vi "AlliGator Special Controls Update.vi"(8 "error in (no error)":errorcluster, 9 "AlliGator Settings List Element":T1, 11 "VI Refnum":refnum<vi>) -> (0 "Error Out":errorcluster, 1 "Message":string, 2 "VI Name":string, 3 "VI Refnum (dup)":refnum<vi>)   [LabVIEW 2021, in "AlliGator Settings.lvlib"]
doc: "Handles update of some Settings controls & indicators as a result of settings changes."
uses:
  AlliGator Settings.lvlib
  AlliGator Settings List.ctl
  Variant/Variant to Data/Variant to Boolean.vi
  Variant/Variant to Data/Variant to DBL.vi
  Variant/Variant to Data/Variant to [String].vi
  Variant/Variant to Data/Variant to I32.vi
  Variant/Variant to Data/Variant to Data.lvlib
  Utilities/Utilities.lvlib
panel:
  in  "Operations Order":u16(ring) caption="Order" items=["Revert", "Smoothen", "Straighten", "Extrapolate", "Normalize", "Background subtraction", "Shift"]
  # "see the AlliGator License on the block diagram (Ctrl+E or Window:Show Block Diagram)"
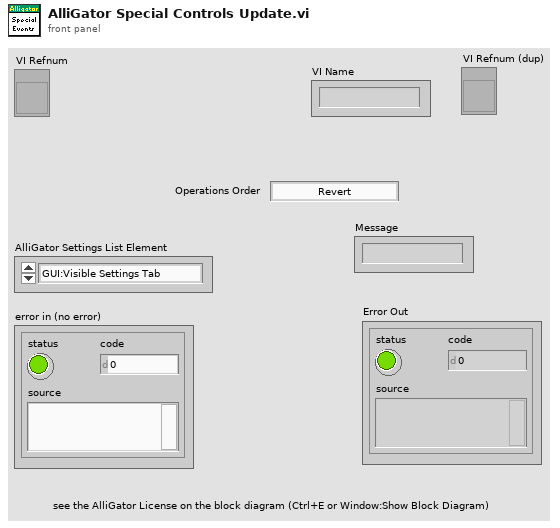
[diagram p1: front panel]
types:
  T1 = typedef "AlliGator Settings.lvlib/AlliGator Settings List.ctl" = enum16{"GUI:Visible Settings Tab", "GUI:Last Run Version", "Source Image:Use Image Histogram for Contrast", "Source Image:Low Count Pixels Rejection Options", "Source Image:High Count Pixels Rejection Options", "Source Image:Use Image Brightness", "Source Image:Blend Overlay with Image Background", "Source Image:Use Fixed ROI Diameter", "Source Image:ROI Diameter", "Source Image:ROI Center Color", "Source Image:Peak Threshold", "Source Image:Intensity Threshold", "Source Image:Image Binning Options", "Source Image:Image Smoothing Options", "Source Image:Image Histogram Active", "Source Image:Invert Binary Mask", "Source Image:Hot Pixel Removal", "Source Image:Overlay Analyzed ROI Center", "Source Image:Auto-Adjust Contrast", "Source Image:Histogram Lower Percentile", "Source Image:Histogram Upper Percentile", "Source Image:Save Source Image", "Source Image:Scale Bar Options", "Source Image:Image Resolution (Pixel Size)", "Source Image:Flatfield Correction", "Source Image:Show Dead Left Columns Correction", "Source Image:Dead Left Columns Correction", "Source Image:Image Pre-Processing Operations Order", "Source Image:Overlay ROI Median", "Source Image:Median Overlay Color", "Data Information:Gate Width", "Data Information:Nanotime Gate Separation", "Data Information:Macrotime Gate Separation", "Data Information:Gate Step", "Data Information:# Gates", "Data Information:Gate Image Exposure", "Data Information:Gate Image Integration", "Data Information:Gates to Skip", "Data Information:Gates to Keep", "Data Information:Define Gates to", "Data Information:Channel Name", "Data Information:Available Channel Names", "Data Information:Channel Arithmetic", "Data Information:Background File Subtraction", "Data Information:Background File", "Data Information:Background Scaling Factor", "Data Information:Background Pile-up Correction", "Data Information:Background Pixel Well Capacity", "Data Information:Laser Period", "Data Information:SYNC Period", "Data Information:Pile-up Correction", "Data Information:Pixel Well Capacity", "Data Information:Dataset Scaling Factor", "Fluorescence Decay_Decay Pre-Processing:Reverse Gates", "Fluorescence Decay_Decay Pre-Processing:Verbose Decay Pre-Processing", "Fluorescence Decay_Decay Pre-Processing:Use Decay Pre-Processing", "Fluorescence Decay_Decay Pre-Processing:Background Subtraction", "Fluorescence Decay_Decay Pre-Processing:Background Definition Range", "Fluorescence Decay_Decay Pre-Processing:Baseline Subtraction Method", "Fluorescence Decay_Decay Pre-Processing:Decay Pre-Processing Operations Order", "Fluorescence Decay_Decay Pre-Processing:Smoothing Parameter", "Fluorescence Decay_Decay Pre-Processing:Shift Decay", "Fluorescence Decay_Decay Pre-Processing:Decay Shift Parameters", "Fluorescence Decay_Decay Pre-Processing:Fold Decay", "Fluorescence Decay_Decay Pre-Processing:# Folds", "Fluorescence Decay_Decay Pre-Processing:1-Normalize Decay", "Fluorescence Decay_Decay Pre-Processing:[0-1]-Normalize Decay", "Fluorescence Decay_Decay Pre-Processing:Smoothen Decay", "Fluorescence Decay_Decay Pre-Processing:Extrapolate Decay", "Fluorescence Decay_Decay Pre-Processing:Use Periodicity", "Fluorescence Decay_Decay Pre-Processing:Use Cursors", "Fluorescence Decay_Decay Pre-Processing:Tail Fraction", "Fluorescence Decay_Decay Pre-Processing:Head Fraction", "Fluorescence Decay_Decay Pre-Processing:Additional Points", "Fluorescence Decay_Decay Pre-Processing:Straighten Decay", "Fluorescence Decay_Decay Pre-Processing:Constant Background", "Fluorescence Decay_Decay Pre-Processing:Pixel-Normalize Decay", "Fluorescence Decay_Advanced Analysis:Extract IRF instead of Decay", "Fluorescence Decay_Advanced Analysis:IRF Extraction Options", "Fluorescence Decay_Advanced Analysis:IRF Optimization Options", "Fluorescence Decay_Advanced Analysis:Square Pulse Options", "Fluorescence Decay_Advanced Analysis:IRF Order", "Fluorescence Decay_Advanced Analysis:IRF Time Constants", "Fluorescence Decay_Advanced Analysis:Wavelet Analysis Options", "Fluorescence Decay_Advanced Analysis:Average Lifetime Options", "Fluorescence Decay_Fit Options:Fit Options", "Fluorescence Decay_Fit Options:Use Legacy Fitting Approach", "Fluorescence Decay_Fit Options:Use Data Information Laser Period", "Fluorescence Decay_Fit Parameters:Displayed Fit Parameters", "Fluorescence Decay_Fit Parameters:Fit Parameter Constraints", "Fluorescence Decay_Fit Parameters:Export Tabulated Results", "Fluorescence Decay_Fit Parameters:MLE Baseline Offset Type", "Fluorescence Decay_Fit Parameters:MLE Baseline Offset", "Fluorescence Decay_Fit Parameters:Guess Parameter Names", "Fluorescence Decay_Fit Parameters:Guess Parameter Values", "Fluorescence Decay_Fit Parameters:Guess Parameters Options", "Fluorescence Decay_Styles:Show Last Decay Only", "Fluorescence Decay_Styles:Decay Graph Color Array", "Fluorescence Decay:Decay Graph Active", "Fluorescence Decay Statistics:Min Peak Value", "Fluorescence Decay Statistics:Reject Low Decay Peak Pixels", "Fluorescence Decay Statistics:Reject High Decay Peak Pixels", "Fluorescence Decay Statistics:Max Peak Value", "Time Traces:Use File Timestamp", "Time Traces:Time Step", "Time Traces:Use Intensity Correction File", "Time Traces:Intensity Correction File", "Phasor Plot:Phasor Plot Smoothing Options", "Phasor Plot:Phasor Plot Size", "Phasor Plot:Phasor Plot Graphics Options", "Phasor Plot:Cumulative Phasor Plot", "Phasor Plot:Use Phasor Brightness", "Phasor Plot:Blend Overlay with Phasor Background", "Phasor Plot:Save Phasor Plot", "Phasor Plot:Show References", "Phasor Plot:Phasor Ratio Decay Range", "Phasor Plot:Exponential Fading", "Phasor Plot:Phasor Ratio Reference Colors", "Phasor Plot:Reference Radius", "Phasor Plot:Show Color Map Vertices", "Phasor Plot:Phasor Plot Active", "Phasor Plot:Phasor Ratio Color Map Type", "Phasor Plot:Phasor Ratio Color Map", "Phasor Plot:Phasor Ratio Display Range", "Phasor Plot:Selected Image ROI(s)", "Phasor Plot:All Image ROIs", "Phasor Plot:Selected Phasor Plot ROI(s)", "Phasor Plot:All Phasor Plot ROIs", "Phasor Plot:Phasor Ratio Color-Coded Quantity", "Phasor Plot:Store Phasor Harmonics", "Phasor Plot:Draw Reference Segment", "Phasor Plot:User-Defined Quantity", "Phasor Graph:Phasor Frequency", "Phasor Graph:Phasor Ratio Type", "Phasor Graph:Pixel-level Phasor Computation", "Phasor Graph:Save Phasor Graph", "Phasor Graph:Phasor Graph Active", "Phasor Graph:Phasor SDV Options", "Phasor Calibration:Use Backup Calibration if needed", "Phasor Graph:Define Shortest Lifetime as", "Phasor Calibration:Backup Calibration Type", "Phasor Calibration:Calibration Type", "Phasor Calibration:Calibration Lifetime", "Phasor Calibration:Calibration Map Algorithm", "Single-Exponential Phasor Locus (SEPL):Gate Parameters", "Single-Exponential Phasor Locus (SEPL):User-defined Gate", "Single-Exponential Phasor Locus (SEPL):User-defined IRF", "Single-Exponential Phasor Locus (SEPL):Phasor Parameters", "Single-Exponential Phasor Locus (SEPL):Decay & IRF Parameters", "Single-Exponential Phasor Locus (SEPL):Display Parameters", "Lifetime Analysis:Decay Analysis Parameters", "Lifetime Analysis:Lifetime Map Active", "Plugins:Python Settings", "Miscellaneous:Verbose Mode", "Miscellaneous:Beep after Script", "Miscellaneous:Saved Image File Format", "Miscellaneous:Exported Gate Image Settings", "Miscellaneous:Include Loading in Timing", "Miscellaneous:Verbose Settings Mode", "Miscellaneous:Histogram Options", "Miscellaneous:Beep on Error", "Miscellaneous:# Logical Processors Used", "Miscellaneous:ROI Description Max Characters", "Miscellaneous:Verbose Error Mode", "Miscellaneous:Transparent Mask Color"}
  T2 = enum16{"Controls & Indicators", "Controls", "Indicators"}
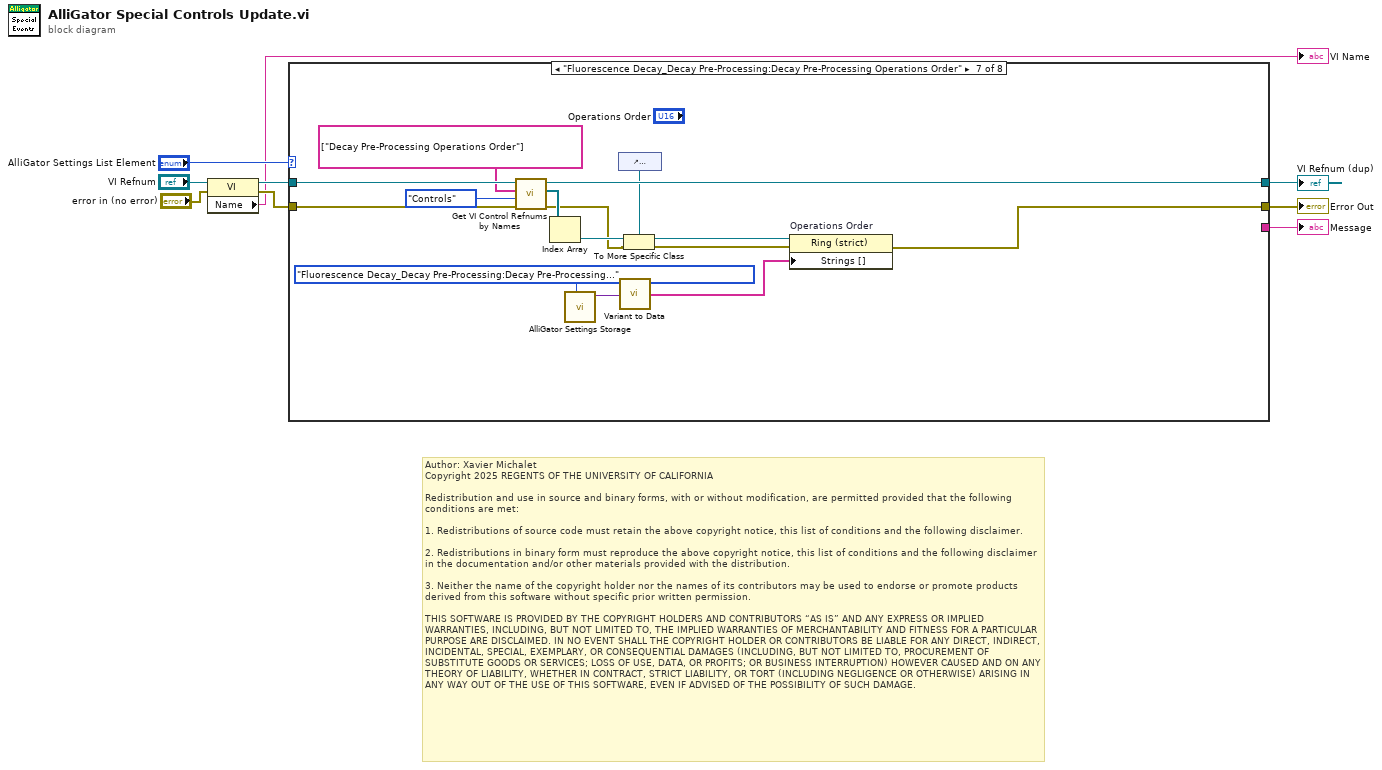
[diagram p0: block diagram]
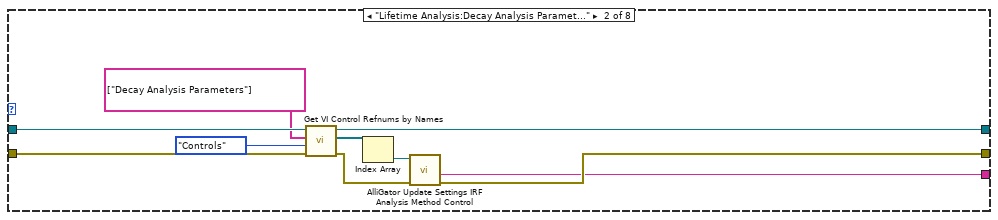
[diagram p3: hidden frame]
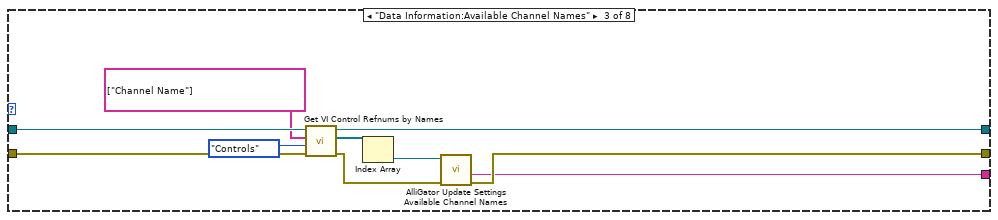
[diagram p4: hidden frame]
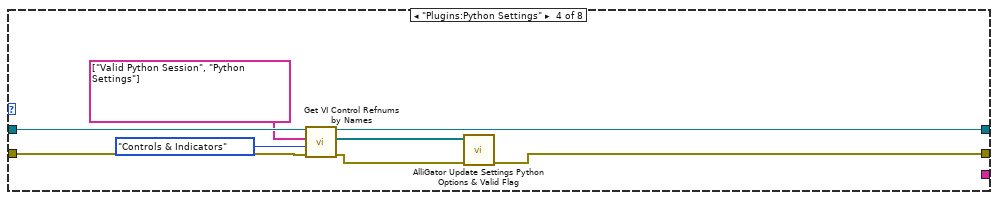
[diagram p5: hidden frame]
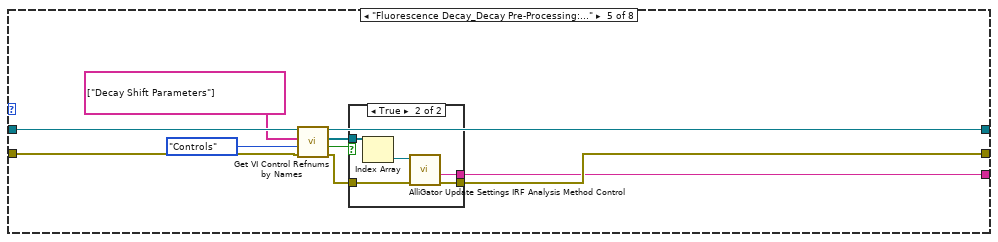
[diagram p6: hidden frame]
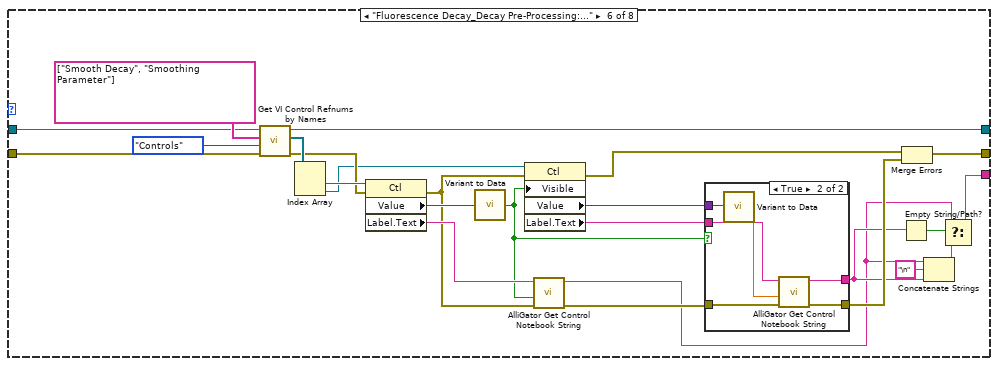
[diagram p8: hidden frame]
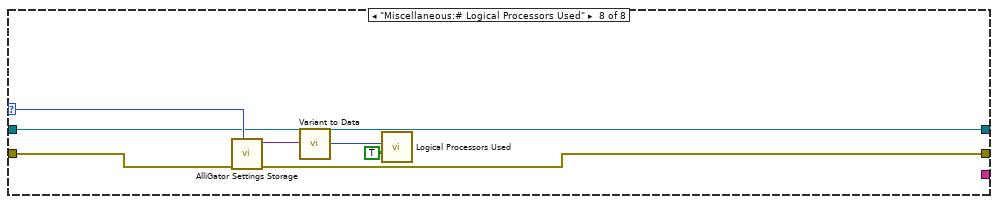
[diagram p10: hidden frame]
diagram:
  # "Author: Xavier Michalet\nCopyright 2025 REGENTS OF THE UNIVERSITY OF CALIFORNIA\n\nRedistribution and use in source and binary forms, with or without modification, are permitted provided that the following conditions are met:\n\n1. Redistributions of source code must retain the above copyright notice, this list of conditions and the following disclaimer.\n\n2. Redistributions in binary form must reproduce the above copyright notice, this list of conditions and the following disclaimer in the documentation and/or other materials provided with the distribution.\n\n3. Neither the name of the copyright holder nor the names of its contributors may be used to endorse or promote products derived from this software without specific prior written permission.\n\nTHIS SOFTWARE IS PROVIDED BY THE COPYRIGHT HOLDERS AND CONTRIBUTORS “AS IS” AND ANY EXPRESS OR IMPLIED WARRANTIES, INCLUDING, BUT NOT LIMITED TO, THE IMPLIED WARRANTIES OF MERCHANTABILITY AND FITNESS FOR A PARTICULAR PURPOSE ARE DISCLAIMED. IN NO EVENT SHALL THE COPYRIGHT HOLDER OR CONTRIBUTORS BE LIABLE FOR ANY DIRECT, INDIRECT, INCIDENTAL, SPECIAL, EXEMPLARY, OR CONSEQUENTIAL DAMAGES (INCLUDING, BUT NOT LIMITED TO, PROCUREMENT OF SUBSTITUTE GOODS OR SERVICES; LOSS OF USE, DATA, OR PROFITS; OR BUSINESS INTERRUPTION) HOWEVER CAUSED AND ON ANY THEORY OF LIABILITY, WHETHER IN CONTRACT, STRICT LIABILITY, OR TORT (INCLUDING NEGLIGENCE OR OTHERWISE) ARISING IN ANY WAY OUT OF THE USE OF THIS SOFTWARE, EVEN IF ADVISED OF THE POSSIBILITY OF SUCH DAMAGE."
  n1 = property class="VI"(reference="VI Refnum", error in="error in (no error)") -> (reference out=w6:refnum<vi>, error out=w4:errorcluster, "Name"=→"VI Name":string)
  n2 = case shown="\"Fluorescence Decay_Decay Pre-Processing:Decay Pre-Processing Operations Order\"" "AlliGator Settings List Element" {
    selector: "AlliGator Settings List Element" -> [_ _ _ _ _ _ _ w109]
    tunnel: w6 -> [w11 w21 w31 w39 w49 w77 w102 w103]
    tunnel: w4 -> [w10 w20 w30 w38 w48 w76 w101 w106]
    tunnel: [w11 w19 w29 w37 w47 w75 w100 w103] -> w2
    tunnel: [w10 w18 w28 w36 w46 w63 w88 w107] -> w8
    tunnel: [_ w17 w27 _ w45 w58 _ _] -> w1
    frame "GUI:Visible Settings Tab", Default {
    }
    frame "Lifetime Analysis:Decay Analysis Parameters" {
      n3 = call "Get VI Control Refnums by Names.vi"("error in"=w20, "Selection"=T2."Controls", "Control Labels"=string[] ["Decay Analysis Parameters"], "VI  Ref"=w21) -> ("error out"=w13:errorcluster, "Ctl Refnums"=w14:refnum<vi>[], "VI  Ref (out)"=w19:refnum<vi>)  [unwired: 4 in, 1 out]
      n4 = Index Array(array=w14) -> (element=w12:refnum<vi>)  [unwired: 1 in]
      n5 = call "AlliGator Update Settings IRF Analysis Method Control.vi"("error in (no error)"=w13, "IRF Analysis Method Refnum"=w12) -> ("error out"=w18:errorcluster, "Message"=w17:string)  [unwired: 8 in]
    }
    frame "Data Information:Available Channel Names" {
      n6 = call "Get VI Control Refnums by Names.vi"("error in"=w30, "Selection"=T2."Controls", "Control Labels"=string[] ["Channel Name"], "VI  Ref"=w31) -> ("error out"=w22:errorcluster, "Ctl Refnums"=w24:refnum<vi>[], "VI  Ref (out)"=w29:refnum<vi>)  [unwired: 4 in, 1 out]
      n7 = Index Array(array=w24) -> (element=w23:refnum<vi>)  [unwired: 1 in]
      n8 = call "AlliGator Update Settings Available Channel Names.vi"("error in (no error)"=w22, "Gate Name Refnum"=w23) -> ("error out"=w28:errorcluster, "Message"=w27:string)  [unwired: 8 in]
    }
    frame "Plugins:Python Settings" {
      n9 = call "Get VI Control Refnums by Names.vi"("error in"=w38, "Selection"=T2."Controls & Indicators", "Control Labels"=string[] ["Valid Python Session", "Python Settings"], "VI  Ref"=w39) -> ("error out"=w33:errorcluster, "Ctl Refnums"=w32:refnum<vi>[], "VI  Ref (out)"=w37:refnum<vi>)  [unwired: 4 in, 1 out]
      n10 = call "AlliGator Update Settings Python Options & Valid Flag.vi"("error in (no error)"=w33, "Ctl Refnums"=w32) -> ("error out"=w36:errorcluster)  [unwired: 9 in]
    }
    frame "Fluorescence Decay_Decay Pre-Processing:Shift Decay" {
      n11 = call "Get VI Control Refnums by Names.vi"("error in"=w48, "Selection"=T2."Controls", "Control Labels"=string[] ["Decay Shift Parameters"], "VI  Ref"=w49) -> ("error out"=w41:errorcluster, "All Ctls found?"=w40:bool, "Ctl Refnums"=w42:refnum<vi>[], "VI  Ref (out)"=w47:refnum<vi>)  [unwired: 4 in]
      n12 = case shown="True" w40 {
        tunnel: w42 -> [_ w55]
        tunnel: w41 -> [w50 w54]
        tunnel: [w50 w52] -> w46
        tunnel: [_ w51] -> w45
        frame False {
        }
        frame True {
          n13 = Index Array(array=w55) -> (element=w53:refnum<vi>)  [unwired: 1 in]
          n14 = call "AlliGator Update Settings IRF Analysis Method Control.vi"("error in (no error)"=w54, "IRF Analysis Method Refnum"=w53) -> ("error out"=w52:errorcluster, "Message"=w51:string)  [unwired: 8 in]
        }
      }
    }
    frame "Fluorescence Decay_Decay Pre-Processing:Smoothing Parameter" {
      n15 = call "Get VI Control Refnums by Names.vi"("error in"=w76, "Selection"=T2."Controls", "Control Labels"=string[] ["Smooth Decay", "Smoothing Parameter"], "VI  Ref"=w77) -> ("error out"=w69:errorcluster, "Ctl Refnums"=w78:refnum<vi>[], "VI  Ref (out)"=w75:refnum<vi>)  [unwired: 4 in, 1 out]
      n16 = Index Array(array=w78) -> (element #1=w70:refnum<vi>, element #2=w68:refnum<vi>)  [unwired: 2 in]
      n17 = property class="Ctl"(reference=w70, error in=w69) -> (error out=w71:errorcluster, "Value"=w74:variant, "Label.Text"=w72:string)  [unwired: 1 out]
      n18 = call-poly "Variant to Data.vi"("Variant"=w74) -> ("Value"=w67:bool)  [unwired: 8 in]
      n19 = property class="Ctl"(reference=w68, error in=w71, "Visible"=w67) -> (error out=w73:errorcluster, "Value"=w66:variant, "Label.Text"=w65:string)  [unwired: 1 out]
      n20 = call "AlliGator Get Control Notebook String.vi"("error in (no error)"=w71, "Value"=w67, "Control Label"=w72) -> ("error out"=w64:errorcluster, "Notebook String"=w56:string)  [unwired: 7 in]
      n21 = case shown="True" w67 {
        tunnel: w66 -> [_ w87]
        tunnel: w65 -> [_ w85]
        tunnel: w64 -> [w81 w84]
        tunnel: [w81 w83] -> w62
        tunnel: [_ w82] -> w57
        frame False {
        }
        frame True {
          n22 = call-poly "Variant to Data.vi"("Variant"=w87) -> ("Value"=w86:dbl)  [unwired: 8 in]
          n23 = call "AlliGator Get Control Notebook String.vi"("error in (no error)"=w84, "Value"=w86, "Control Label"=w85) -> ("error out"=w83:errorcluster, "Notebook String"=w82:string)  [unwired: 7 in]
        }
      }
      n24 = Empty String/Path?(string/path=w57) -> (empty?=w60:bool)
      n25 = Merge Errors(w73, w62) -> (w63:errorcluster)
      n26 = Concatenate Strings(w56, "\n" ("string"), w57) -> (w59:string)
      n27 = Select(t=w56, s=w60, f=w59) -> (s? t:f=w58:string)
    }
    frame "Fluorescence Decay_Decay Pre-Processing:Decay Pre-Processing Operations Order" {
      n28 = call "Get VI Control Refnums by Names.vi"("error in"=w101, "Selection"=T2."Controls", "Control Labels"=string[] ["Decay Pre-Processing Operations Order"], "VI  Ref"=w102) -> ("error out"=w94:errorcluster, "Ctl Refnums"=w98:refnum<vi>[], "VI  Ref (out)"=w100:refnum<vi>)  [unwired: 4 in, 1 out]
      n29 = Index Array(array=w98) -> (element=w99:refnum<vi>)  [unwired: 1 in]
      n30 = call "AlliGator Settings Storage.vi"("AlliGator Settings List"=AlliGator_Settings_List."Fluorescence Decay_Decay Pre-Processing:Decay Pre-Processing Operations Order") -> ("Variant Data out"=w90:variant)  [unwired: 9 in, 1 out]
      n31 = control-ref of="Operations Order"() -> (w92:refnum<vi>)
      n32 = call-poly "Variant to Data.vi"("Variant"=w90) -> ("String Array"=w89:string[])  [unwired: 8 in]
      n33 = To More Specific Class(target class=w92, reference=w99, error in=w94) -> (specific class reference=w95:refnum<vi>, error out=w93:errorcluster)
      n34 = property on="Operations Order" class="Ring (strict)"(reference=w95, error in=w93, "Strings []"=w89) -> (error out=w88:errorcluster)  [unwired: 1 out]
    }
    frame "Miscellaneous:# Logical Processors Used" {
      n35 = call "AlliGator Settings Storage.vi"("AlliGator Settings List"=w109, "Error In"=w106) -> ("Error Out"=w107:errorcluster, "Variant Data out"=w108:variant)  [unwired: 8 in]
      n36 = call-poly "Variant to Data.vi"("Variant"=w108) -> ("Value"=w105:i32)  [unwired: 8 in]
      n37 = call "Logical Processors Used.vi"("Set/Get (F)"=TRUE, "# Logical Processor Used"=w105) -> ()  [unwired: 4 in, 1 out]
    }
  }
  "Error Out" <- w8
  "VI Refnum (dup)" <- w2
  "Message" <- w1
